vi "7L24_perso.vi"() -> ()   [LabVIEW 2010]
panel:
  in  "Cc":dbl
  in  "T":dbl
  out "Cc init":dbl
  out "T init":dbl
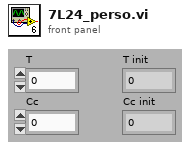
[diagram p1: front panel]
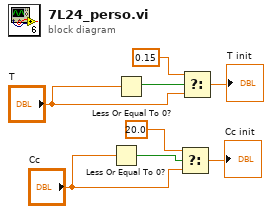
[diagram p0: block diagram]
diagram:
  n1 = Less Or Equal To 0?(x="Cc") -> (x <= 0?=w5:bool)
  n2 = Less Or Equal To 0?(x="T") -> (x <= 0?=w4:bool)
  n3 = Select(t=20.0 ("cas vrai"), s=w5, f="Cc") -> (s? t:f=→"Cc init":dbl)
  n4 = Select(t=0.15 ("cas vrai"), s=w4, f="T") -> (s? t:f=→"T init":dbl)
